vi "Read Light Stack.vi"(8 "error in (no error)":errorcluster, 11 "PLC in":refnum<class "PLC.lvclass">) -> (0 "error out":errorcluster, 2 "Light Stack":refnum<class "Light Stack.lvclass">, 3 "PLC out":refnum<class "PLC.lvclass">)   [LabVIEW 2018, in "PLC.lvlib" / "PLC.lvclass"]
uses:
  PLC.lvclass
  PPLs/PLC/Light Stack/Light Stack.lvlibp/Light Stack.lvclass
  PLC.lvclass/PLC.ctl
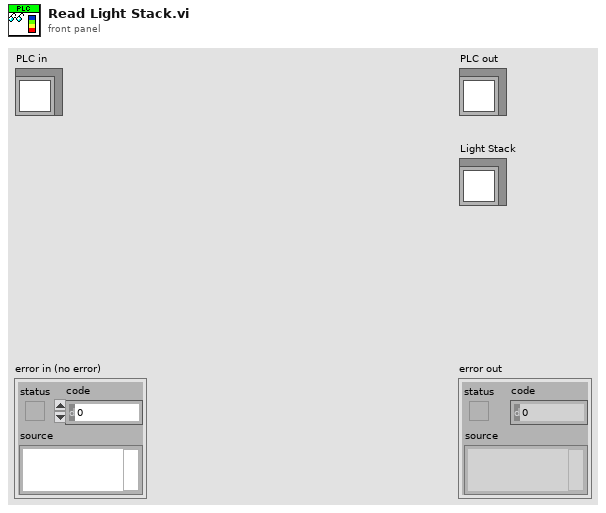
[diagram p1: front panel]
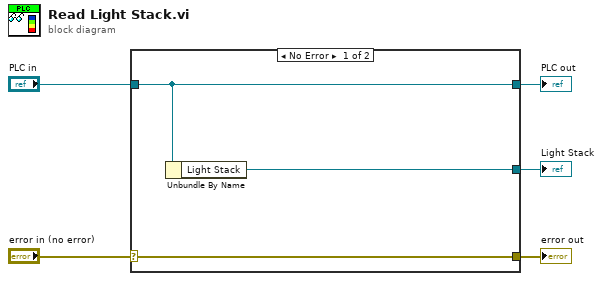
[diagram p0: block diagram]
diagram:
  n1 = case shown="No Error" "error in (no error)" {
    selector: "error in (no error)" -> [w8 w9]
    tunnel: [w8 w9] -> w4
    tunnel: [w7 w10] -> w2
    tunnel: "PLC in" -> [w7 w10]
    tunnel: [w6 _] -> w1
    frame No Error {
      n2 = Unbundle By Name(w7) -> ("Light Stack"=w6:refnum<class "Light Stack.lvclass">)
    }
    frame Error {
    }
  }
  "error out" <- w4
  "PLC out" <- w2
  "Light Stack" <- w1
